vi "niFPGA Shift 2 Saturate (I64 to 32).vi"(2 "I64 input":i64 format="%08x") -> (6 "saturated I32 output":i32 format="%.0x")   [LabVIEW 2017]
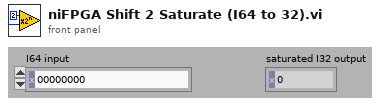
[diagram p1: front panel]
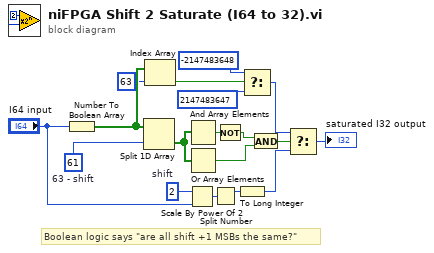
[diagram p0: block diagram]
diagram:
  w18 = i8 2  # shift
  w17 = i8 61  # 63 - shift
  # "Boolean logic says \"are all shift +1 MSBs the same?\""
  n1 = Number To Boolean Array(number="I64 input") -> (Boolean array=w14:bool[])
  n2 = Split 1D Array(array=w14, index=w17) -> (second subarray=w15:bool[])  [unwired: 1 out]
  n3 = Index Array(array=w14, index=63) -> (element=w12:bool)
  n4 = Scale By Power Of 2(n=w18, x="I64 input") -> (x*2^n=w3:i64)
  n5 = And Array Elements(Boolean array=w15) -> (logical AND=w8:bool)
  n6 = Or Array Elements(Boolean array=w15) -> (logical OR=w6:bool)
  n7 = Split Number(x=w3) -> (hi(x)=w2:u32)  [unwired: 1 out]
  n8 = Not(x=w8) -> (.not. x?=w7:bool)
  n9 = To Long Integer(number=w2) -> (32bit integer=w1:i32)
  n10 = Select(t=-2147483648, s=w12, f=2147483647) -> (s? t:f=w4:i32)
  n11 = And(x=w7, y=w6) -> (x .and. y?=w5:bool)
  n12 = Select(t=w4, s=w5, f=w1) -> (s? t:f=→"saturated I32 output":i32)
